vi "SDG60CreateArbWaveform.vi"(5 "WFM (Column) Number":i32, 6 "Array WFM":i16[](array[numeric])=[1000, 2000, 3000, 4000, 5000, 6000, 7000, 8000], 7 "WFM Length":i32=15, 8 "error in (no error)":errorcluster, 9 "Timeout (40000 ms)":u32=40000, 10 "Waveform Name (\"wave1\")":string="wave1", 11 "VISA resource name":refnum<visa-resource-name>="USB0::0xF4EC::0x1101::SDG6XEBC5R0119::INSTR") -> (0 "error out":errorcluster, 3 "VISA resource name out":refnum<visa-resource-name>)   [LabVIEW 2018]
doc: "Creates and saves an arbitrary (user-defined) waveform in non-volatile memory, then selects it for output."
uses:
  <vilib>/Utility/file.llb/Read From Spreadsheet File (I64).vi
panel:
  out "WFM to arr time":dbl
  out "Arr to str time":dbl
  out "Upload time":dbl
  out "Total time":dbl
  out "Attempts":i32
  in  "WFM Source":u16(ring) items=["Single file", "Split files", "Array"]
  in  "WFM Path":path=path "C:/Data/_SoftDevelopment/SDG6000/data67107840.txt"
  # "Need to set name to be number. not string"
  # "Same vi as with suppliers example,\nbut incorrect negativ case removed.\nInstead calculating twos complement\nexplicitly for negative values.\nThe input range for ARB data is\n-32767..+32767"
  # "C1 hardcoded as needs to have a channel\nassigned to be uploaded. \nCan then be selected for either channel"
  # "Max  20E6 (decimal)"
  # "Need to reset device (*RST) to upload long (?) wavelength from PC to device\nFor now can't see another way to clear memory."
  # "Upon overwrite of name with new WFM, still needs to be selected\notherwise will still use old WFM. If WFM has been selected, and then gets deleted off \nC drive, will still output WFM on that channel"
  # "Testing uploads of large WFMS.\n8M: All ok, can have 2 separate WFMs on 2 channels and upload more\n16M: Can have 2 separate WFMs on 2 channels, storage space limits 3rd upload\n          of 16M points, but can upload 8M and switch fine between them all. Can't\n          upload an overwriting 16M point WFM when 2 already saved.\n20M: Can have 20M on both channels, but then no storage space to upload, need to delete\n          old waveform. Upon deletion, can upload 20M and select fine. \n          Could not do this yesterday, so may require more investigation.\nIf too large a waveform is uploaded, generator will crash requiring manual power cycle\n                 Can have 20E6 WFM on one channel\n                  Can't have 20E6 on both channels - freezes when selecting 2nd WFM"
  # "If storage full, will beep on \nmachine-say storage full, \nbut not give any error through \nlabview. Waveform won't ovewrite\nothers when uploading"
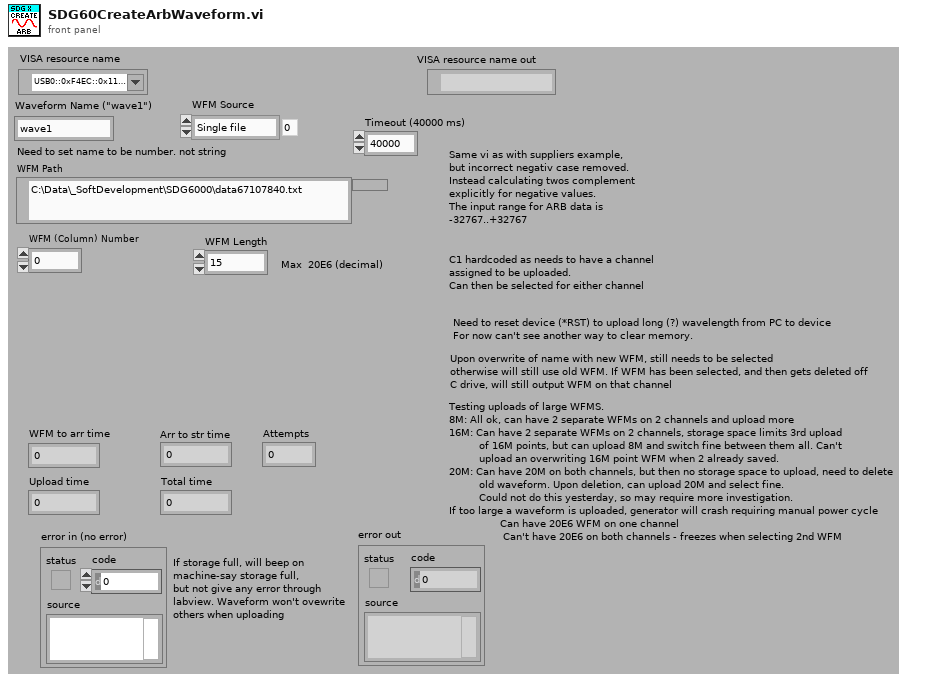
[diagram p1: front panel]
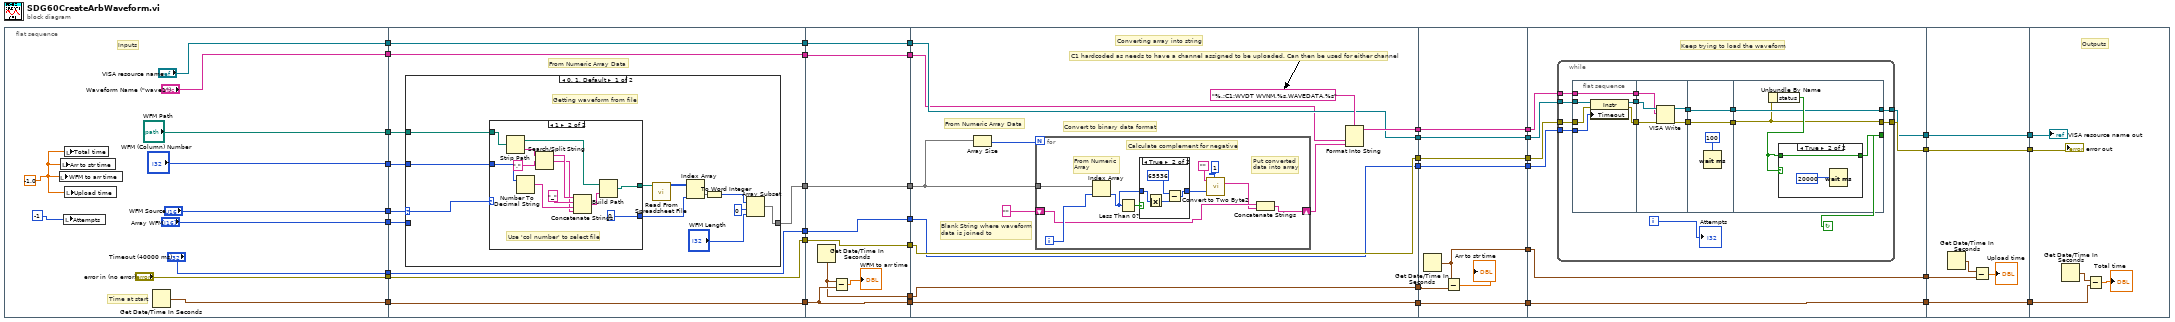
[diagram p0: block diagram]
diagram:
  n1 = flat-sequence {
    tunnel: ["WFM Source"] -> w41
    tunnel: ["Array WFM"] -> w40
    tunnel: ["WFM Path"] -> w39
    tunnel: ["WFM (Column) Number"] -> w38
    tunnel: ["VISA resource name"] -> w37
    tunnel: ["Waveform Name (\"wave1\")"] -> w36
    tunnel: ["error in (no error)"] -> w35
    tunnel: ["Timeout (40000 ms)"] -> w34
    tunnel: [w44] -> w33
    tunnel: w41 -> [w62]
    tunnel: w40 -> [w61]
    tunnel: [w60] -> w32
    tunnel: w39 -> [w59]
    tunnel: w38 -> [w58]
    tunnel: [w57] -> w30
    tunnel: w37 -> [w57]
    tunnel: [w56] -> w28
    tunnel: w36 -> [w56]
    tunnel: [w55] -> w26
    tunnel: w35 -> [w55]
    tunnel: [w54] -> w24
    tunnel: w34 -> [w54]
    tunnel: [w53] -> w22
    tunnel: w33 -> [w53]
    tunnel: w32 -> [w96]
    tunnel: [w96] -> w31
    tunnel: w30 -> [w95]
    tunnel: [w95] -> w29
    tunnel: w28 -> [w94]
    tunnel: [w94] -> w27
    tunnel: w26 -> [w90]
    tunnel: [w90] -> w25
    tunnel: w24 -> [w91]
    tunnel: [w91] -> w23
    tunnel: w22 -> [w92]
    tunnel: [w92] -> w21
    tunnel: [w89] -> w1
    tunnel: w31 -> [w104]
    tunnel: [w103] -> w20
    tunnel: [w102] -> w18
    tunnel: [w101] -> w16
    tunnel: [w100] -> w14
    tunnel: w29 -> [w102]
    tunnel: w27 -> [w99]
    tunnel: w25 -> [w101]
    tunnel: w23 -> [w100]
    tunnel: w21 -> [w98]
    tunnel: [w98] -> w12
    tunnel: [w97] -> w2
    tunnel: w1 -> [w97]
    tunnel: w20 -> [w131]
    tunnel: [w131] -> w19
    tunnel: w18 -> [w130]
    tunnel: [w130] -> w17
    tunnel: w16 -> [w129]
    tunnel: [w129] -> w15
    tunnel: w14 -> [w128]
    tunnel: [w128] -> w13
    tunnel: w12 -> [w124]
    tunnel: [w124] -> w11
    tunnel: [w126] -> w4
    tunnel: w2 -> [w125]
    tunnel: [w135] -> w10
    tunnel: [w134] -> w8
    tunnel: w19 -> [w139]
    tunnel: w17 -> [w138]
    tunnel: w15 -> [w137]
    tunnel: w13 -> [w136]
    tunnel: w11 -> [w133]
    tunnel: [w133] -> w6
    tunnel: w4 -> [w132]
    tunnel: [w132] -> w3
    tunnel: w10 -> [w181]
    tunnel: [w181] -> w9
    tunnel: w8 -> [w180]
    tunnel: [w180] -> w7
    tunnel: w6 -> [w178]
    tunnel: [w178] -> w5
    tunnel: w3 -> [w177]
    tunnel: w9 -> [w186]
    tunnel: w7 -> [w185]
    tunnel: w5 -> [w182]
    frame #0 {
      w43 = -1.0
      # "Inputs"
      # "Time at start"
      n2 = local write "WFM to arr time"(w43) -> ()
      n3 = local write "Arr to str time"(w43) -> ()
      n4 = local write "Attempts"(-1) -> ()
      n5 = local write "Total time"(w43) -> ()
      n6 = local write "Upload time"(w43) -> ()
      n7 = Get Date/Time In Seconds() -> (seconds since 1Jan1904=w44:timestamp)
    }
    frame #1 {
      # "From Numeric Array Data"
      n8 = case shown="0, 1, Default" w62 {
        selector: w62 -> [w70 _]
        tunnel: [w65 w88] -> w60
        tunnel: w61 -> [_ w88]
        tunnel: w59 -> [w64 _]
        tunnel: w58 -> [w63 _]
        frame 0, 1, Default {
          # "Getting waveform from file"
          n9 = case shown="1" w70 {
            tunnel: w64 -> [w75 w87]
            tunnel: w63 -> [w74 w84]
            tunnel: [w75 w77] -> w68
            tunnel: [w74 0 ("x")] -> w67
            frame 0, Default {
              # "File contains multiple wfms"
            }
            frame 1 {
              # "Use 'col number' to select file"
              n10 = Strip Path(path=w87) -> (stripped path=w79:path, name=w85:string)
              n11 = Number To Decimal String(number=w84) -> (decimal integer string=w81:string)  [unwired: 1 in]
              n12 = Search/Split String(string=w85, search string/char (-)=".") -> (substring before match=w83:string, match + rest of string=w80:string)  [unwired: 1 in, 1 out]
              n13 = Concatenate Strings(w83, "_", w81, w80) -> (w78:string)
              n14 = Build Path(base path=w79, name or relative path=w78) -> (appended path=w77:path)
            }
          }
          n15 = call-poly <vilib>:"Read From Spreadsheet File.vi"("file path (dialog if empty)"=w68) -> ("all rows"=w69:i64[][])  [unwired: 6 in, 4 out]
          n16 = Index Array(array=w69, index (col)=w67) -> (element=w66:i64[])  [unwired: 1 in]
          n17 = To Word Integer(number=w66) -> (16bit integer=w73:i16[])
          n18 = Array Subset(array=w73, index=0 ("x"), length="WFM Length") -> (w65:i16[])
        }
        frame 2 {
          # "Arbitrary Numeric Waveform Data"
        }
      }
    }
    frame #2 {
      n19 = Get Date/Time In Seconds() -> (seconds since 1Jan1904=w89:timestamp)
      n20 = Subtract(x=w89, y=w92) -> (x-y=→"WFM to arr time":dbl)
    }
    frame #3 {
      # "Converting array into string"
      # "Blank String where waveform\ndata is joined to"
      # "C1 hardcoded as needs to have a channel assigned to be uploaded. Can then be used for either channel"
      # "From Numeric Array Data"
      # "Convert to binary data format"
      n21 = Array Size(array=w104) -> (size(s)=w107:i32)
      n22 = for {
        N: w107 -> [_]
        shift-right: [w112] -> w105
        shift-left: "" -> [w111]
        tunnel: w104 -> [w109]
        i -> [w116]
        # "Calculate complement for negative"
        # "From Numeric\nArray"
        # "Put converted\ndata into array"
        n23 = Index Array(array=w109, index=w116) -> (element=w114:i16)
        n24 = Less Than 0?(x=w114) -> (x < 0?=w115:bool)
        n25 = case shown="True" w115 {
          tunnel: w114 -> [w119 w120]
          tunnel: [w119 w123] -> w113
          frame False {
          }
          frame True {
            n26 = Absolute Value(x=w120) -> (abs(x)=w121:i16)
            n27 = Subtract(x=65536, y=w121) -> (x-y=w123:i32)
          }
        }
        n28 = call "Convert to Two Byte2.vi"("Input Method (0:String)"=u16 1, "Input Number"=w113, "Numeric String"="") -> ("Output String"=w110:string)  [unwired: 8 in]
        n29 = Concatenate Strings(w111, w110) -> (w112:string)
      }
      n30 = Format Into String(format string="%.;C1:WVDT WVNM,%s,WAVEDATA,%s", w99, w105) -> (resulting string=w103:string)  [unwired: 2 in, 1 out]
    }
    frame #4 {
      n31 = Get Date/Time In Seconds() -> (seconds since 1Jan1904=w126:timestamp)
      n32 = Subtract(x=w126, y=w125) -> (x-y=→"Arr to str time":dbl)
    }
    frame #5 {
      # "Keep trying to load the waveform"
      n33 = while {
        tunnel: w139 -> [w154]
        tunnel: w138 -> [w153]
        tunnel: w137 -> [w152]
        tunnel: [w151] -> w135
        tunnel: [w150] -> w134
        tunnel: w136 -> [w140]
        i -> [w146]
        stop <- w149 continue-if-true
        n34 = flat-sequence {
          tunnel: w154 -> [w160]
          tunnel: w152 -> [w157]
          tunnel: w153 -> [w159]
          tunnel: [w158] -> w143
          tunnel: [w156] -> w142
          tunnel: [w160] -> w141
          tunnel: w140 -> [w155]
          tunnel: [w161] -> w148
          tunnel: [w162] -> w147
          tunnel: w143 -> [w164]
          tunnel: w142 -> [w165]
          tunnel: w141 -> [w163]
          tunnel: w148 -> [w166]
          tunnel: w147 -> [w167]
          tunnel: [w167] -> w145
          tunnel: [w166] -> w144
          tunnel: [w170] -> w150
          tunnel: [w169] -> w151
          tunnel: [w171] -> w149
          tunnel: w145 -> [w170]
          tunnel: w144 -> [w169]
          frame #0 {
            n35 = property class="Instr"(reference=w159, error in=w157, "Timeout"=w155) -> (reference out=w158:refnum<visa-resource-name>, error out=w156:errorcluster)
          }
          frame #1 {
            n36 = VISA Write(VISA resource name=w164, write buffer=w163, error in (no error)=w165) -> (VISA resource name out=w162:refnum<visa-resource-name>, error out=w161:errorcluster)  [unwired: 1 out]
          }
          frame #2 {
            n37 = Wait (ms)(milliseconds to wait=100 ("x")) -> ()  [unwired: 1 out]
          }
          frame #3 {
            n38 = Unbundle By Name(w169) -> ("status"=w172:bool)
            n39 = case shown="True" w172 {
              tunnel: w172 -> [w173 w174]
              tunnel: [w173 w174] -> w171
              frame False {
              }
              frame True {
                n40 = Wait (ms)(milliseconds to wait=20000 ("x")) -> ()  [unwired: 1 out]
              }
            }
          }
        }
        "Attempts" <- w146
      }
    }
    frame #6 {
      n41 = Get Date/Time In Seconds() -> (seconds since 1Jan1904=w179:timestamp)
      n42 = Subtract(x=w179, y=w177) -> (x-y=→"Upload time":dbl)
    }
    frame #7 {
      # "Outputs"
      n43 = Get Date/Time In Seconds() -> (seconds since 1Jan1904=w184:timestamp)
      n44 = Subtract(x=w184, y=w182) -> (x-y=→"Total time":dbl)
      "VISA resource name out" <- w185
      "error out" <- w186
    }
  }
